vi "CheckIfVIPartOfG#IDE.vi"(1 "Path":path, 5 "error in (no error)":errorcluster) -> (15 "PartOfG#IDE?":bool, 19 "error out":errorcluster)   [LabVIEW 2020, in "G#Installer.lvlib"]
uses:
  G#Installer.lvlib
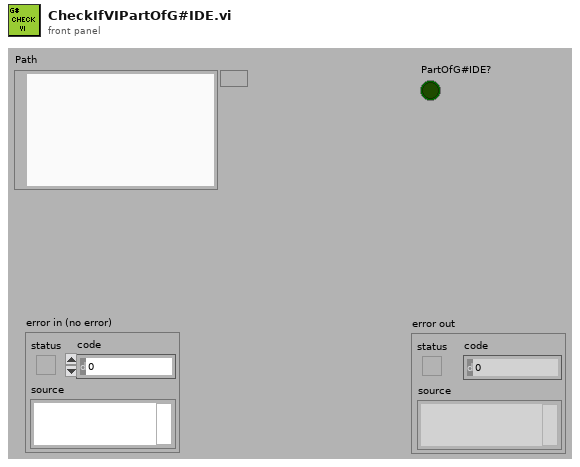
[diagram p1: front panel]
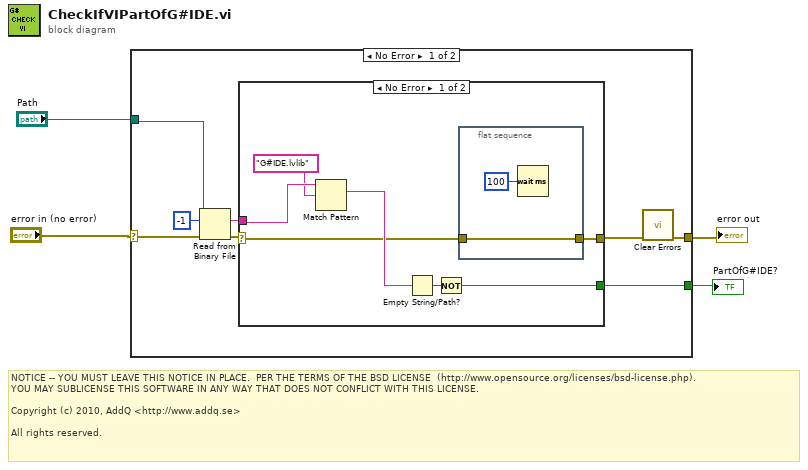
[diagram p0: block diagram]
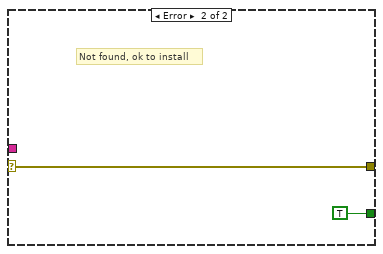
[diagram p2: hidden frame]
diagram:
  # "NOTICE -- YOU MUST LEAVE THIS NOTICE IN PLACE.  PER THE TERMS OF THE BSD LICENSE  (http://www.opensource.org/licenses/bsd-license.php).\nYOU MAY SUBLICENSE THIS SOFTWARE IN ANY WAY THAT DOES NOT CONFLICT WITH THIS LICENSE.\n\nCopyright (c) 2010, AddQ <http://www.addq.se>\n\nAll rights reserved."
  n1 = case shown="No Error" "error in (no error)" {
    selector: "error in (no error)" -> [w12 w24]
    tunnel: "Path" -> [w10 _]
    tunnel: [w6 w24] -> w2
    tunnel: [w7 _] -> w1
    frame No Error {
      n2 = Read from Binary File(8:w12, 10:-1 ("count (1)"), 11:w10) -> (0:w9:errorcluster, 2:w8:string)  [unwired: 3 in, 2 out]
      n3 = case shown="No Error" w9 {
        selector: w9 -> [w14 w22]
        tunnel: w8 -> [w19 _]
        tunnel: [w15 TRUE] -> w7
        tunnel: [w13 w22] -> w5
        frame No Error {
          n4 = Match Pattern(string=w19, regular expression="G#IDE.lvlib") -> (match substring=w17:string)  [unwired: 1 in, 3 out]
          n5 = Empty String/Path?(string/path=w17) -> (empty?=w16:bool)
          n6 = Not(x=w16) -> (.not. x?=w15:bool)
          n7 = flat-sequence {
            tunnel: w14 -> [w20]
            tunnel: [w20] -> w13
            frame #0 {
              n8 = Wait (ms)(milliseconds to wait=u32 100) -> ()  [unwired: 1 out]
            }
          }
        }
        frame Error {
          # "Not found, ok to install"
        }
      }
      n9 = call <vilib>:"Clear Errors.vi"("error in (no error)"=w5) -> ("error out"=w6:errorcluster)  [unwired: 5 in, 1 out]
    }
    frame Error {
    }
  }
  "error out" <- w2
  "PartOfG#IDE?" <- w1
